vi "Readmimetype.vi"(8 "error in (no error)":errorcluster, 11 "object in":refnum<class "kernel_info_reply Message.lvclass">) -> (0 "error out":errorcluster, 2 "mimetype":string, 3 "object out":refnum<class "kernel_info_reply Message.lvclass">)   [LabVIEW 2018, in "ClientMessaging.lvlib" / "kernel_info_reply Message.lvclass"]
uses:
  kernel_info_reply Message.lvclass
  kernel_info_reply Message.lvclass/kernel_info_reply Message.ctl
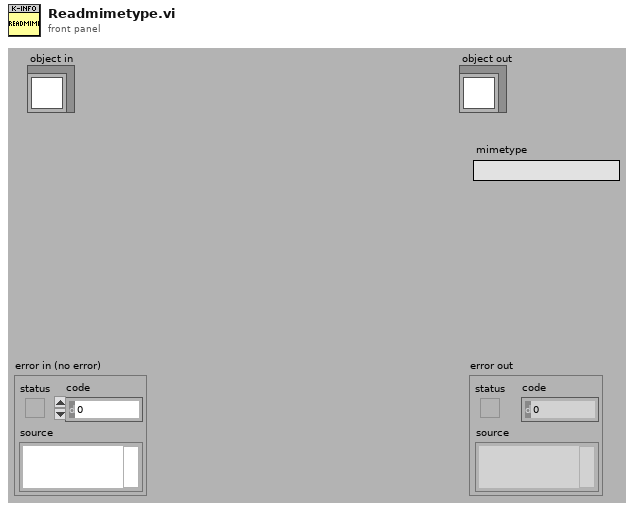
[diagram p1: front panel]
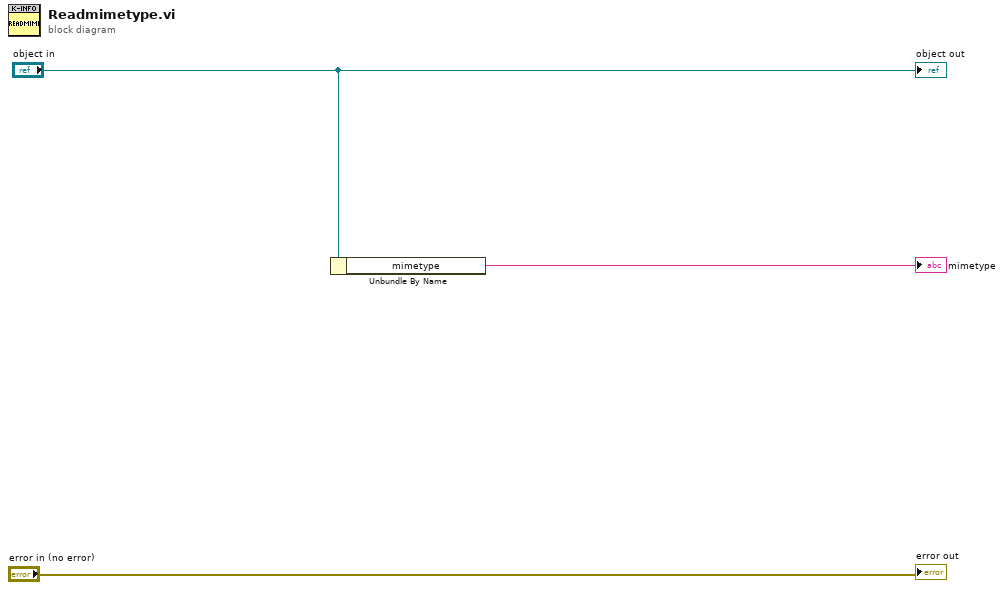
[diagram p0: block diagram]
diagram:
  n1 = Unbundle By Name("object in") -> ("mimetype"=→"mimetype":string)
  "error out" <- "error in (no error)"
  "object out" <- "object in"
